vi "rqcAlice SPI.Send Raw Value.vi"(7 "SPI.subSystem":T1=enum."Attenuation.dB", 8 "error in":errorcluster, 10 "value":u16, 11 "Alice FPGA Reference In":refnum<k20>) -> (0 "error out":errorcluster, 3 "Alice FPGA Reference Out":refnum<k20>)   [LabVIEW 2018]
uses:
  Shared/Shared Host Lib/SPI/typedefs/SPI.SubSystem.ctl
  Shared/Shared Host Lib/SPI/typedefs/SPI.FPGA Interface.ctl
  <vilib>/Utility/error.llb/Error Cluster From Error Code.vi
  <vilib>/rvi/errors/niLvFpgaAdjustHostInterfaceError.vi
  <vilib>/rvi/interface/nirviReadWriteControl/nirviReadWriteControl.xnode
  NiFpgaLv.dll
  <vilib>/rvi/interface/Simulation/niFpgaSimulationCallBeginRW.vi
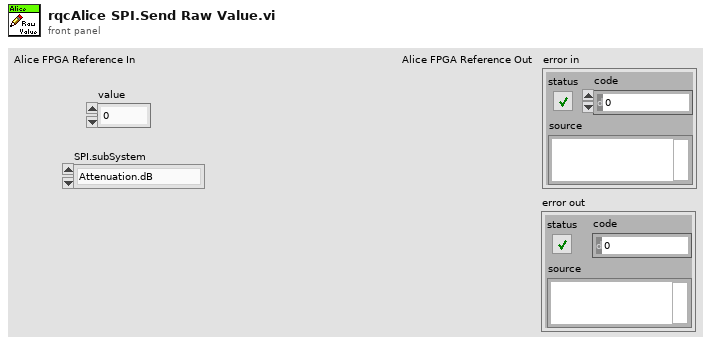
[diagram p1: front panel]
types:
  T1 = typedef "SPI.SubSystem.ctl" = enum8{"N/A", "DelayLine.MSB", "DelayLine.LSB", "Attenuation.dB", "Attenuation.DAC value", "SyncDetector.Offset", "SyncDetector.Comparator", "PM.Value[0]", "PM.Value[1]", "PM.Value[2]", "PM.Value[3]"}
  T2 = typedef "SPI.FPGA Interface.ctl" = refnum<k20>
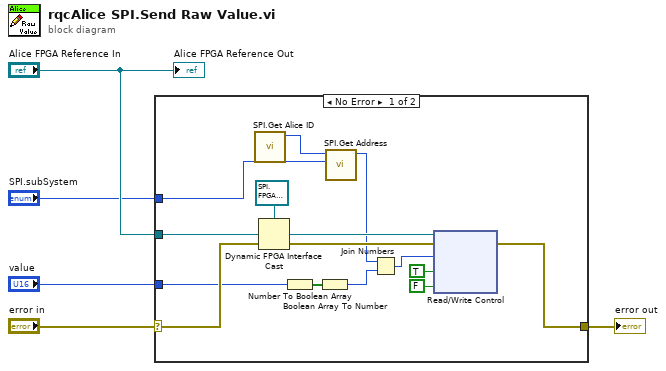
[diagram p0: block diagram]
diagram:
  n1 = case shown="No Error" "error in" {
    selector: "error in" -> [w13 w20]
    tunnel: [w10 w20] -> w4
    tunnel: "Alice FPGA Reference In" -> [w19 _]
    tunnel: "value" -> [w9 _]
    tunnel: "SPI.subSystem" -> [w6 _]
    frame No Error {
      n2 = call "SPI.Get Alice ID.vi"() -> ("Alice.ID"=w12:u8)  [unwired: 11 in]
      n3 = Dynamic FPGA Interface Cast(Session In=T2 refnum ("Type"), Type=w19) -> (Session Out=w14:T2)
      n4 = Number To Boolean Array(number=w9) -> (Boolean array=w8:bool[])
      n5 = Boolean Array To Number(Boolean array=w8) -> (number=w7:u16)
      n6 = call "SPI.Get Address.vi"("SPI.subSystem"=w6, "ID"=w12) -> ("Address"=w11:u16)  [unwired: 9 in]
      n7 = Join Numbers(hi=w11, lo=w7) -> ((hi.lo)=w15:u32)
      n8 = xnode "Read/Write Control"("FPGA VI Reference In"=w14, "error in"=w13, "SPI.data"=w15, "SPI.write"=TRUE ("reset"), "SPI.write"=FALSE ("reset")) -> ("error out"=w10:errorcluster)  [unwired: 1 out]
    }
    frame Error {
    }
  }
  "error out" <- w4
  "Alice FPGA Reference Out" <- "Alice FPGA Reference In"
